vi "Board Player on Board.vi"(1 "Height":i32, 2 "Width":i32, 3 "Player":refnum<class "Player.lvclass">) -> (0 "In Range?":bool)   [LabVIEW 2019, in "Board.lvclass"]
uses:
  Board.lvclass
  Player/Player.lvclass
  Snake/Snake.lvclass
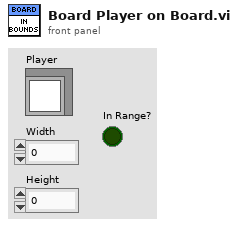
[diagram p1: front panel]
types:
  T1 = typedef "Snake.lvclass/Snake Component STYP.ctl" = cluster{"Direction":T2, "Coordinate":T3}
  T2 = typedef "Direction STYP.ctl" = enum16{"Up", "Down", "Left", "Right"}
  T3 = typedef "Coordinate STYP.ctl" = cluster{"X":i32, "Y":i32}
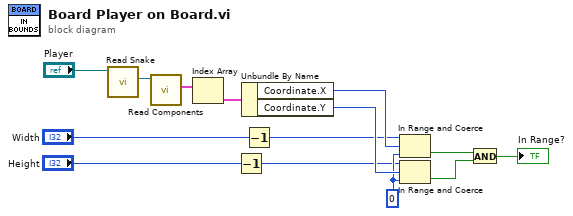
[diagram p0: block diagram]
diagram:
  w6 = 0 ("lower limit")
  n1 = call-dynamic "Read Snake.vi"("Player in"="Player") -> ("Snake.lvclass"=w13:refnum<class "Snake.lvclass">)  [unwired: 8 in, 2 out]
  n2 = call-dynamic "Read Components.vi"("Snake in"=w13) -> ("Components"=w12:T1[])  [unwired: 8 in, 2 out]
  n3 = Index Array(array=w12) -> (element=w11:T1)  [unwired: 1 in]
  n4 = Decrement(x="Height") -> (x-1=w4:i32)
  n5 = Unbundle By Name(w11) -> ("Coordinate.X"=w10:i32, "Coordinate.Y"=w9:i32)
  n6 = Decrement(x="Width") -> (x-1=w5:i32)
  n7 = In Range and Coerce(upper limit=w5, x=w10, lower limit=w6) -> (In Range?=w3:bool)  [unwired: 1 out]
  n8 = In Range and Coerce(upper limit=w4, x=w9, lower limit=w6) -> (In Range?=w2:bool)  [unwired: 1 out]
  n9 = And(x=w3, y=w2) -> (x .and. y?=→"In Range?":bool)
